vi "Save Octree.vi"(1 "Octree node array":T1[](array[typedef]), 2 "Octree file path":path) -> (0 "Error out":errorcluster)   [LabVIEW 2014]
uses:
  Typedefs/TreeNodeBox.ctl
  Typedefs/Quad.ctl
  Typedefs/Quadplane enum.ctl
panel:
  # "PN 23/01/2015"
  # "Vertices"
  # "Edges"
  # "Unit normal"
  # "Plane ident."
  # "Vertices"
  # "Edges"
  # "Unit normal"
  # "Plane ident."
  # "Vertices"
  # "Edges"
  # "Unit normal"
  # "Plane ident."
  # "Vertices"
  # "Edges"
  # "Unit normal"
  # "Plane ident."
  # "Vertices"
  # "Edges"
  # "Unit normal"
  # "Plane ident."
  # "Vertices"
  # "Edges"
  # "Unit normal"
  # "Plane ident."
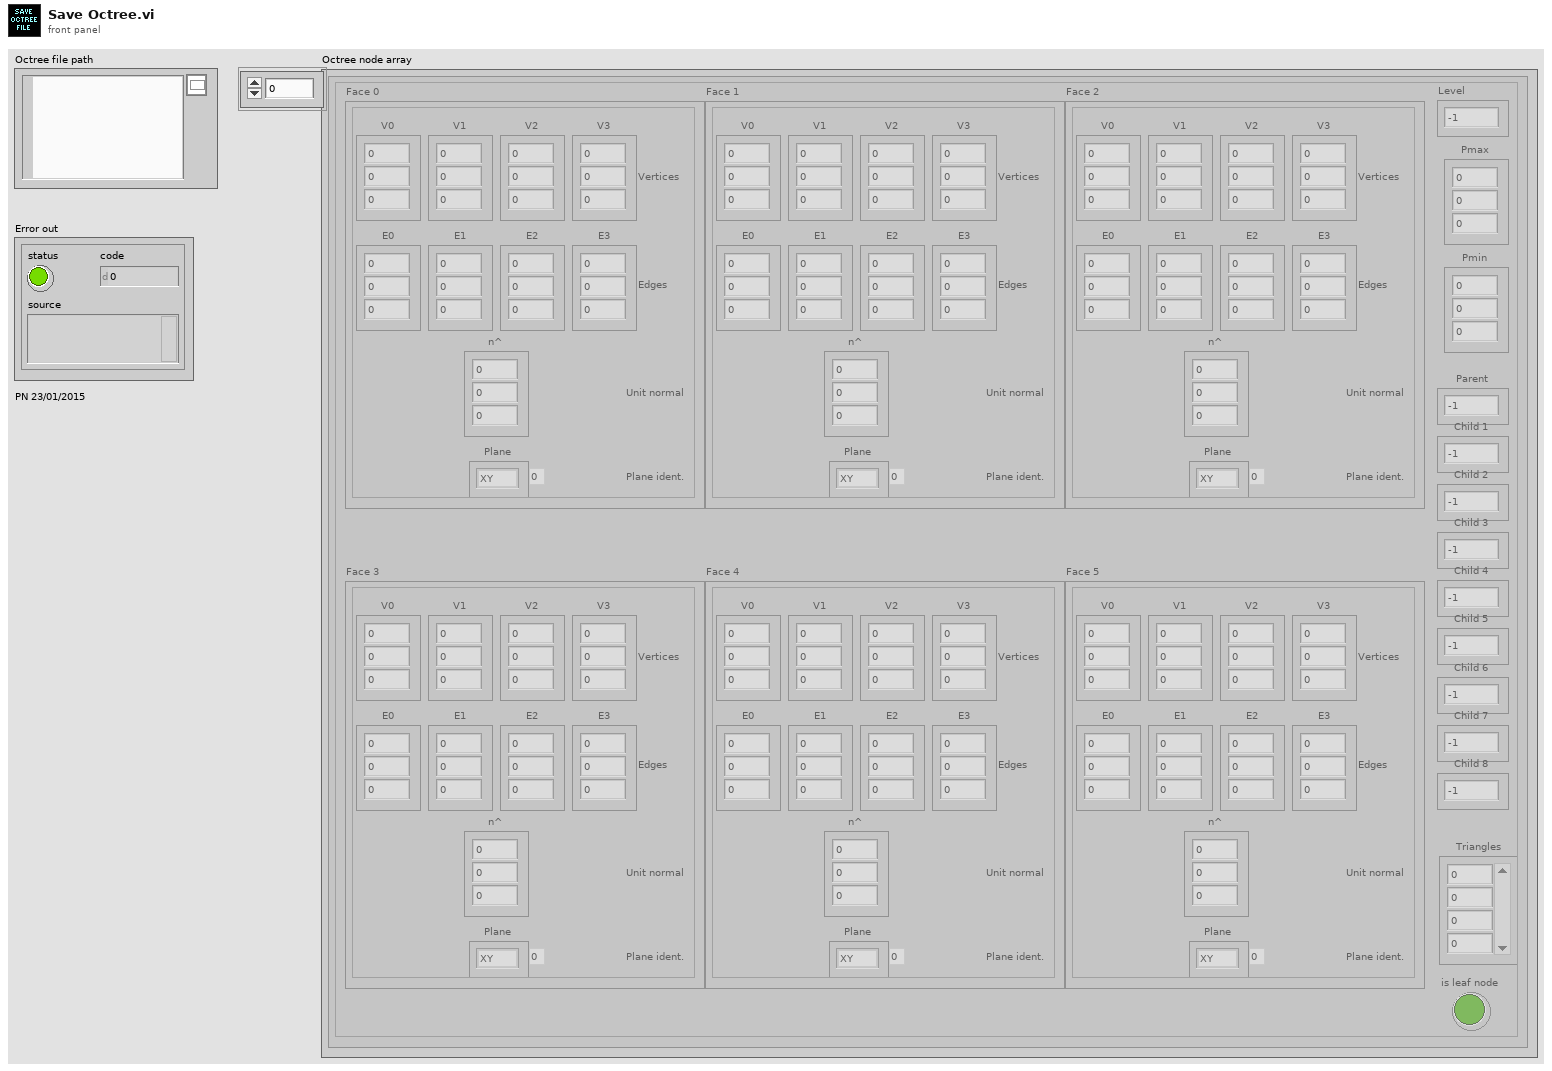
[diagram p1: front panel]
types:
  T1 = typedef "TreeNodeBox.ctl" = cluster{"Face 0":T2, "Face 1":T2, "Face 2":T2, "Face 3":T2, "Face 4":T2, "Face 5":T2, "Level":i32, "Pmax":sgl[], "Pmin":sgl[], "Parent":i32, "Child 1":i32, "Child 2":i32, "Child 3":i32, "Child 4":i32, "Child 5":i32, "Child 6":i32, "Child 7":i32, "Child 8":i32, "Triangles":i32[], "is leaf node":bool}
  T2 = typedef "Quad.ctl" = cluster{"V0":sgl[], "V1":sgl[], "V2":sgl[], "V3":sgl[], "E0":sgl[], "E1":sgl[], "E2":sgl[], "E3":sgl[], "n^":sgl[], "Plane":T3}
  T3 = typedef "Quadplane enum.ctl" = enum8{"XY", "XZ", "YZ", "-XY", "-XZ", "-YZ"}
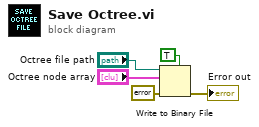
[diagram p0: block diagram]
diagram:
  n1 = Write to Binary File(file (use dialog)="Octree file path", data="Octree node array", error in=errorcluster {"status"=FALSE, "code"=0, "source"=""} ("error in (no error)"), 5:TRUE ("prepend array or string size? (T)")) -> (error out=→"Error out":errorcluster)  [unwired: 2 in, 2 out]
